vi "ex5-9.vi"() -> ()   [LabVIEW 2014]
uses:
  <vilib>/NXT/Subs/MotorOutput.ctl
  <vilib>/NXT/Block Support/NXT_OutputPort.ctl
  <vilib>/NXT/Block Support/NXT_InputPort.ctl
  <vilib>/NXT/Dual Mode Library/Motors/ResetMotor.vi
  <vilib>/NXT/Dual Mode Library/Motors/Rotation.vi
  <vilib>/NXT/Dual Mode Library/Motors/MotorOn.vi
  <vilib>/NXT/Dual Mode Library/Sensors/Touch_Pressed.vi
  <vilib>/NXT/Dual Mode Library/Motors/MotorBrake.vi
panel:
  out "Numeric":dbl
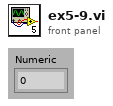
[diagram p1: front panel]
types:
  T1 = typedef "MotorOutput.ctl" = u8
  T2 = typedef "LVHSConnector.ctl" = refnum<class "BrickReference.lvclass">
  T3 = typedef "NXT_InputPort.ctl" = u32
  T4 = typedef "NXT_OutputPort.ctl" = u8
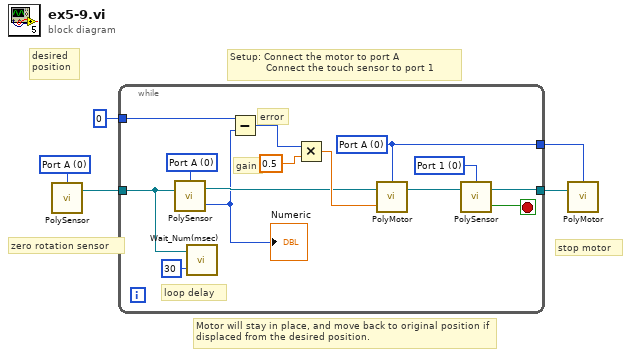
[diagram p0: block diagram]
diagram:
  w5 = T1 0 items=["Port A", "Port B", "Port C", "All Ports"] ("Output Port")
  # "Setup: Connect the motor to port A\n            Connect the touch sensor to port 1"
  # "zero rotation sensor"
  # "desired\nposition"
  # "stop motor"
  # "Motor will stay in place, and move back to original position if displaced from the desired position."
  n1 = call-poly <vilib>:"PolySensor.vi"("Port (All Ports)"=w5) -> ("NXT/EV3"=w4:T2)  [unwired: 1 in, 2 out]
  n2 = while {
    tunnel: 0 ("RotationCount") -> [w17]
    tunnel: [w14] -> w3
    tunnel: w4 -> [w9]
    tunnel: [w13] -> w2
    stop <- w12 stop-if-true
    w7 = T3 0 items=["Port 1", "Port 2", "Port 3", "Port 4"] ("Port (Port 1)")
    w10 = T4 0 items=["Port A", "Port B", "Port C"] ("Output Port (Port A)")
    w14 = T1 0 items=["Port A", "Port B", "Port C", "All Ports"] ("Output Port")
    # "gain"
    # "error"
    # "loop delay"
    n3 = call-poly <vilib>:"PolySensor.vi"("NXT/EV3"=w9, "Port (Port A)"=w10) -> ("Angle of Rotation"=w6:i32, "NXT/EV3"=w11:T2)  [unwired: 1 out]
    "Numeric" <- w6
    n4 = call <vilib>:"Wait_Num(msec).vi"("Time (100 msec)"=u32 30 ("milliseconds to wait"), "NXT/EV3"=w9) -> ()  [unwired: 2 in, 1 out]
    n5 = Subtract(x=w17, y=w6) -> (x-y=w19:i32)
    n6 = Multiply(x=w19, y=0.5) -> (x*y=w15:dbl)
    n7 = call-poly <vilib>:"PolyMotor.vi"("Power (75)"=w15, "NXT/EV3"=w11, "Output Port (All Ports)"=w14) -> ("NXT/EV3"=w16:T2)  [unwired: 1 out]
    n8 = call-poly <vilib>:"PolySensor.vi"("NXT/EV3"=w16, "Port (Port 1)"=w7) -> ("Yes / No"=w12:bool, "NXT/EV3"=w13:T2)  [unwired: 1 out]
  }
  n9 = call-poly <vilib>:"PolyMotor.vi"("NXT/EV3"=w2, "Port (All Ports)"=w3) -> ()  [unwired: 3 out]
